vi "Autonomous Independent.vi"   [LabVIEW 2014]
doc: "This VI is called when autonomous begins, and will automatically be terminated when autonomous ends. You can carry out timed or sensor driven robot movement independently without needing to return to the caller."
uses:
  ChassisLib/ChassisLib.lvlib
  LiftLib/LiftLib.lvlib
  LatchLib/LatchLib.lvlib
  IntakeLib/IntakeLib.lvlib
  PusherLib/PusherLib.lvlib
  GateLib/GateLib.lvlib
panel:
  # "Be sure to right-click and choose Data Operations>>Make Current Value default if you want to save the array values with the VI"
types:
  T1 = enum16{"open", "replace", "create", "open or create", "replace or create", "replace or create with confirmation"}
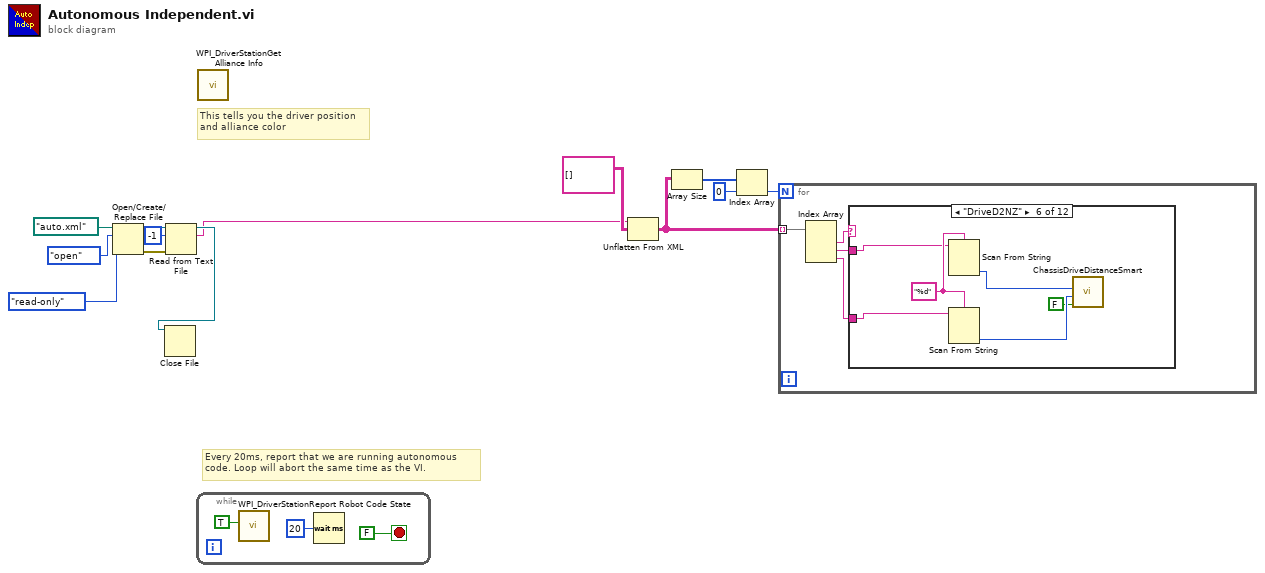
[diagram p0: block diagram]
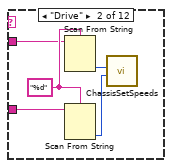
[diagram p3: hidden frame]
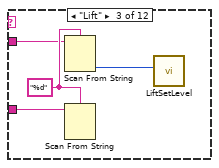
[diagram p4: hidden frame]
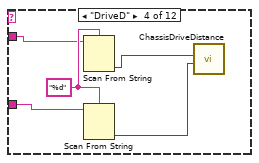
[diagram p5: hidden frame]
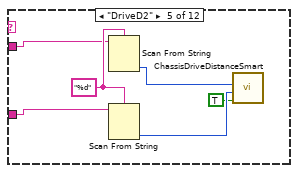
[diagram p6: hidden frame]
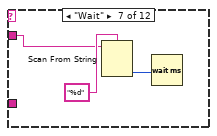
[diagram p7: hidden frame]
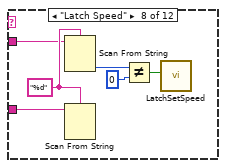
[diagram p8: hidden frame]
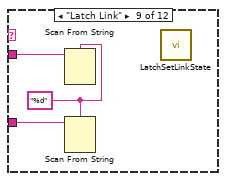
[diagram p9: hidden frame]
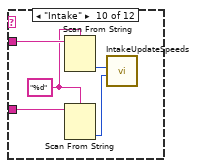
[diagram p10: hidden frame]
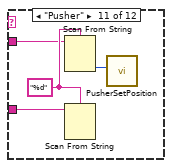
[diagram p11: hidden frame]
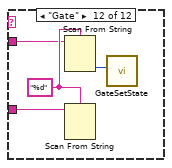
[diagram p12: hidden frame]
diagram:
  # "Every 20ms, report that we are running autonomous\ncode. Loop will abort the same time as the VI."
  # "This tells you the driver position\nand alliance color"
  n1 = Open/Create/Replace File(file path (use dialog)=path "/auto.xml" ("file (use dialog)"), operation (0:open)=T1."open", access (0:read/write)=enum16{"read/write", "read-only", "write-only"}."read-only") -> (refnum out=w10:refnum<file>, error out=w11:errorcluster)  [unwired: 3 in, 1 out]
  n2 = Read from Text File(file (use dialog)=w10, count=-1, error in=w11) -> (refnum out=w8:refnum<file>, text=w2:string)  [unwired: 1 in, 2 out]
  n3 = Close File(refnum=w8) -> ()  [unwired: 1 in, 2 out]
  n4 = while {
    stop <- FALSE stop-if-true
    n5 = call <vilib>:"WPI_DriverStationReport Robot Code State.vi"("Autonomous"=TRUE) -> ()  [unwired: 10 in, 1 out]
    n6 = Wait (ms)(milliseconds to wait=u32 20) -> ()  [unwired: 1 out]
  }
  n7 = call <vilib>:"WPI_DriverStationGet Alliance Info.vi"() -> ()  [unwired: 12 out]
  n8 = Unflatten From XML(xml string=w2, type=string[][] []) -> (value=w3:string[][])  [unwired: 1 in, 1 out]
  n9 = Array Size(array=w3) -> (size(s)=w6:i32[])
  n10 = Index Array(array=w6, index=0) -> (element=w4:i32)
  n11 = for {
    N: w4 -> [_]
    tunnel: w3 -> [w20] mode=indexing
    n12 = Index Array(array=w20) -> (element #1=w19:string, element #2=w17:string, element #3=w18:string)  [unwired: 3 in]
    n13 = case shown="\"DriveD2NZ\"" w19 {
      tunnel: w18 -> [_ w21 w27 w32 w38 w44 _ w53 w57 w61 w65 w69]
      tunnel: w17 -> [_ w22 w28 w33 w39 w45 w48 w54 w58 w63 w66 w70]
      frame "False", Default {
      }
      frame "Drive" {
        w25 = "%d" ("format string")
        n14 = Scan From String(format string=w25, input string=w22) -> (output 1=w24:i32)  [unwired: 3 in, 3 out]
        n15 = Scan From String(format string=w25, input string=w21) -> (output 1=w23:i32)  [unwired: 3 in, 3 out]
        n16 = call "ChassisSetSpeeds.vi"("DriveSpeedRight"=w23, "DriveSpeedLeft"=w24) -> ()  [unwired: 10 in]
      }
      frame "Lift" {
        w29 = "%d" ("format string")
        n17 = Scan From String(format string=w29, input string=w28) -> (output 1=w26:i32)  [unwired: 3 in, 3 out]
        n18 = Scan From String(format string=w29, input string=w27) -> ()  [unwired: 4 in, 3 out]
        n19 = call "LiftSetLevel.vi"("Index"=w26) -> ()  [unwired: 11 in]
      }
      frame "DriveD" {
        w34 = "%d" ("format string")
        n20 = Scan From String(format string=w34, input string=w33) -> (output 1=w31:i32)  [unwired: 3 in, 3 out]
        n21 = Scan From String(format string=w34, input string=w32) -> (output 1=w30:i32)  [unwired: 3 in, 3 out]
        n22 = call "ChassisDriveDistance.vi"("RightDist"=w30, "LeftDist"=w31) -> ()  [unwired: 9 in, 1 out]
      }
      frame "DriveD2" {
        w40 = "%d" ("format string")
        n23 = Scan From String(format string=w40, input string=w39) -> (output 1=w37:i32)  [unwired: 3 in, 3 out]
        n24 = Scan From String(format string=w40, input string=w38) -> (output 1=w36:i32)  [unwired: 3 in, 3 out]
        n25 = call "ChassisDriveDistanceSmart.vi"("Zero"=TRUE, "DriveRight"=w36, "DriveLeft"=w37) -> ()  [unwired: 9 in]
      }
      frame "DriveD2NZ" {
        w46 = "%d" ("format string")
        n26 = Scan From String(format string=w46, input string=w45) -> (output 1=w43:i32)  [unwired: 3 in, 3 out]
        n27 = Scan From String(format string=w46, input string=w44) -> (output 1=w42:i32)  [unwired: 3 in, 3 out]
        n28 = call "ChassisDriveDistanceSmart.vi"("Zero"=FALSE, "DriveRight"=w42, "DriveLeft"=w43) -> ()  [unwired: 9 in]
      }
      frame "Wait" {
        n29 = Scan From String(format string="%d", input string=w48) -> (output 1=w47:i32)  [unwired: 3 in, 3 out]
        n30 = Wait (ms)(milliseconds to wait=w47) -> ()  [unwired: 1 out]
      }
      frame "Latch Speed" {
        w55 = "%d" ("format string")
        n31 = Scan From String(format string=w55, input string=w54) -> (output 1=w52:i32)  [unwired: 3 in, 3 out]
        n32 = Scan From String(format string=w55, input string=w53) -> ()  [unwired: 4 in, 3 out]
        n33 = Not Equal?(x=w52, y=0) -> (x != y?=w50:bool)
        n34 = call "LatchSetSpeed.vi"("LatchLatchState"=w50) -> ()  [unwired: 11 in]
      }
      frame "Latch Link" {
        w56 = "%d" ("format string")
        n35 = Scan From String(format string=w56, input string=w58) -> ()  [unwired: 4 in, 3 out]
        n36 = Scan From String(format string=w56, input string=w57) -> ()  [unwired: 4 in, 3 out]
        n37 = call "LatchSetLinkState.vi"() -> ()  [unwired: 12 in]
      }
      frame "Intake" {
        w62 = "%d" ("format string")
        n38 = Scan From String(format string=w62, input string=w63) -> (output 1=w60:i32)  [unwired: 3 in, 3 out]
        n39 = Scan From String(format string=w62, input string=w61) -> (output 1=w59:i32)  [unwired: 3 in, 3 out]
        n40 = call "IntakeUpdateSpeeds.vi"("IntakeLeftRollerSpeed"=w59, "IntakeRightRollerSpeed"=w60) -> ()  [unwired: 10 in]
      }
      frame "Pusher" {
        w67 = "%d" ("format string")
        n41 = Scan From String(format string=w67, input string=w66) -> (output 1=w64:i32)  [unwired: 3 in, 3 out]
        n42 = Scan From String(format string=w67, input string=w65) -> ()  [unwired: 4 in, 3 out]
        n43 = call "PusherSetPosition.vi"("index"=w64) -> ()  [unwired: 11 in]
      }
      frame "Gate" {
        w71 = "%d" ("format string")
        n44 = Scan From String(format string=w71, input string=w70) -> (output 1=w68:i32)  [unwired: 3 in, 3 out]
        n45 = Scan From String(format string=w71, input string=w69) -> ()  [unwired: 4 in, 3 out]
        n46 = call "GateSetState.vi"("GateCylState"=w68) -> ()  [unwired: 11 in]
      }
    }
  }
